vi "Actor Core.vi"(8 "error in":errorcluster, 11 "HIJ Vision Camera App In":refnum<class "HIJ Vision Camera App.lvclass">) -> (0 "error out":errorcluster, 3 "Actor out":refnum<class "Actor.lvclass">)   [LabVIEW 2014, in "HIJ Vision Camera App.lvlib" / "HIJ Vision Camera App.lvclass"]
doc: "(<B>Filename</B>: Actor Framework.lvlib:Actor.lvclass:Actor Core.vi)\n\nReceives messages to the actor, reacts to them, and initiates any error handling that may shut the actor down.\n\nDescendant classes may override this VI to append parallel tasks for the actor to complete while it handles messages. Overrides use the Call Parent Method node."
uses:
  HIJ Vision Camera App.lvclass
  <vilib>/ActorFramework/Actor/Actor.lvclass
  <vilib>/ActorFramework/Actor/Actor.lvclass/Actor.ctl
  <vilib>/ActorFramework/Message Enqueuer/Message Enqueuer.lvclass/Message Enqueuer.ctl
  HIJ Vision Camera App.lvclass/HIJ Vision Camera App.ctl
  HIJ Vision Camera App Dialog/HIJ Vision Camera App Dialog/HIJ Vision Camera App Dialog.lvclass/HIJ Vision Camera App Dialog.ctl
  HIJ Vision Application/HIJ Vision Application Messages/Write WorkDir Msg/Write WorkDir Msg.lvclass/Write WorkDir Msg.ctl
  HIJ Vision Camera App Messages/Write ConfigDir Msg/Write ConfigDir Msg.lvclass/Write ConfigDir Msg.ctl
  HIJ Vision Application/HIJ Vision Application Messages/Write Image Prefix Msg/Write Image Prefix Msg.lvclass/Write Image Prefix Msg.ctl
  HIJ Vision Camera App Messages/Start Aquisition Msg/Start Aquisition Msg.lvclass/Start Aquisition Msg.ctl
  Shared Code/Viewable Actor/ViewableActor Messages/Insert Into SubPanel Msg/Insert Into SubPanel Msg.lvclass/Insert Into SubPanel Msg.ctl
  HIJ Vision Camera App Dialog/HIJ Vision Camera App Dialog/Read Acquire.vi
  HIJ Vision Camera App Dialog/HIJ Vision Camera App Dialog/Read Camera Name.vi
  HIJ Vision Camera App Dialog/HIJ Vision Camera App Dialog/Read Prefix.vi
  HIJ Vision Camera App Dialog/HIJ Vision Camera App Dialog/Read ConfigDir.vi
  HIJ Vision Camera App Dialog/HIJ Vision Camera App Dialog/Read WorkDir.vi
  <vilib>/ActorFramework/Message Enqueuer/Init from Existing Queue.vi
  <vilib>/ActorFramework/Message Enqueuer/Enqueue.vi
  <vilib>/ActorFramework/Message Priority Queue/Priority Enqueue.vi
  <vilib>/ActorFramework/Message Enqueuer/Message Enqueuer.lvclass
  HIJ Vision Application/HIJ Vision Application Messages/Write WorkDir Msg/Write WorkDir Msg.lvclass
  HIJ Vision Camera App Messages/Write ConfigDir Msg/Write ConfigDir Msg.lvclass
  HIJ Vision Application/HIJ Vision Application Messages/Write Image Prefix Msg/Write Image Prefix Msg.lvclass
  HIJ Vision Camera App Messages/Start Aquisition Msg/Start Aquisition Msg.lvclass
  Shared Code/Viewable Actor/ViewableActor Messages/Insert Into SubPanel Msg/Insert Into SubPanel Msg.lvclass
  HIJ Vision Application/HIJ Vision Application/HIJ Vision Application.lvclass
  HIJ Vision Camera App Dialog/HIJ Vision Camera App Dialog/HIJ Vision Camera App Dialog.lvclass
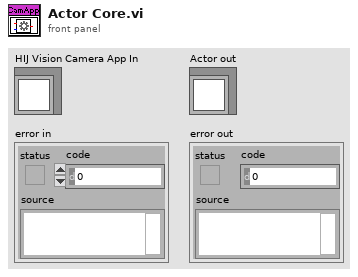
[diagram p1: front panel]
types:
  T1 = typedef "IMAQdx.ctl" = refnum<k21>
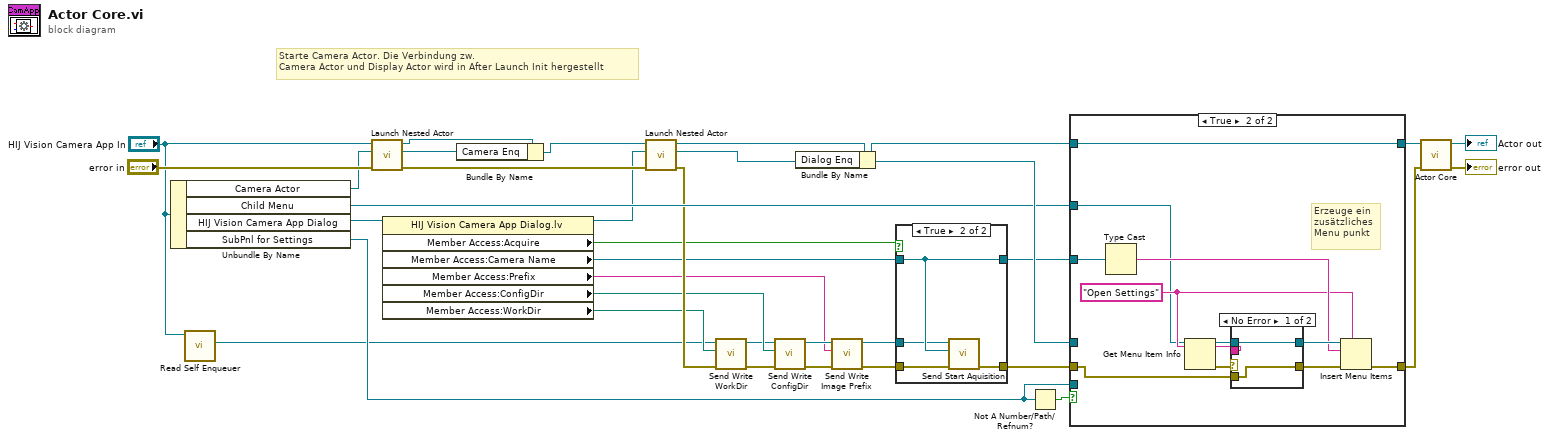
[diagram p0: block diagram]
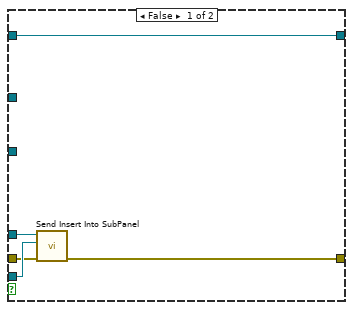
[diagram p3: hidden frame]
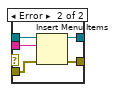
[diagram p4: hidden frame]
diagram:
  # "Starte Camera Actor. Die Verbindung zw.\nCamera Actor und Display Actor wird in After Launch Init hergestellt"
  n1 = Unbundle By Name("HIJ Vision Camera App In") -> ("Camera Actor"=w27:refnum<class "Camera Actor.lvclass">, "Child Menu"=w33:refnum<k9>, "HIJ Vision Camera App Dialog"=w23:refnum<class "HIJ Vision Camera App Dialog.lvclass">, "SubPnl for Settings"=w21:refnum<vi>)
  n2 = call <vilib>:"Read Self Enqueuer.vi"("Actor"="HIJ Vision Camera App In") -> ("Self Enqueuer"=w17:refnum<class "Message Enqueuer.lvclass">)  [unwired: 10 in]
  n3 = call <vilib>:"Launch Nested Actor.vi"("error in (no error)"="error in", "Nested Actor"=w27, "Caller Actor in"="HIJ Vision Camera App In") -> ("error out"=w24:errorcluster, "Nested Actor's Enqueuer"=w26:refnum<class "Message Enqueuer.lvclass">, "Caller Actor out"=w28:refnum<class "HIJ Vision Camera App.lvclass">)  [unwired: 6 in]
  n4 = property class="HIJ Vision Camera App Dialog.lv"(reference=w23) -> (reference out=w19:refnum<class "HIJ Vision Camera App Dialog.lvclass">, "Member Access:Acquire"=w8:bool, "Member Access:Camera Name"=w7:T1, "Member Access:Prefix"=w9:string, "Member Access:ConfigDir"=w16:path, "Member Access:WorkDir"=w18:path)  [unwired: 1 in, 1 out]
  n5 = Bundle By Name(cluster=w28, "Camera Enq"=w26) -> (w25:refnum<class "HIJ Vision Camera App.lvclass">)
  n6 = call <vilib>:"Launch Nested Actor.vi"("error in (no error)"=w24, "Nested Actor"=w19, "Caller Actor in"=w25) -> ("error out"=w32:errorcluster, "Nested Actor's Enqueuer"=w34:refnum<class "Message Enqueuer.lvclass">, "Caller Actor out"=w11:refnum<class "HIJ Vision Camera App.lvclass">)  [unwired: 6 in]
  n7 = call "Send Write WorkDir.vi"("error in (no error)"=w32, "Work Dir"=w18, "Message Enqueuer"=w17) -> ("error out"=w13:errorcluster, "Message Enqueuer out"=w15:refnum<class "Message Enqueuer.lvclass">)  [unwired: 7 in]
  n8 = call "Send Write ConfigDir.vi"("error in (no error)"=w13, "Work Dir"=w16, "Message Enqueuer"=w15) -> ("error out"=w12:errorcluster, "Message Enqueuer out"=w14:refnum<class "Message Enqueuer.lvclass">)  [unwired: 7 in]
  n9 = Bundle By Name(cluster=w11, "Dialog Enq"=w34) -> (w1:refnum<class "HIJ Vision Camera App.lvclass">)
  n10 = call "Send Write Image Prefix.vi"("error in (no error)"=w12, "Prefix"=w9, "Message Enqueuer"=w14) -> ("error out"=w5:errorcluster, "Message Enqueuer out"=w6:refnum<class "Message Enqueuer.lvclass">)  [unwired: 7 in]
  n11 = case shown="True" w8 {
    tunnel: w7 -> [w35 w40]
    tunnel: w6 -> [_ w39]
    tunnel: w5 -> [w36 w38]
    tunnel: [w36 w37] -> w4
    tunnel: [w35 w40] -> w3
    frame False {
    }
    frame True {
      n12 = call "Send Start Aquisition.vi"("error in (no error)"=w38, "Camera"=w40, "Message Enqueuer"=w39) -> ("error out"=w37:errorcluster)  [unwired: 7 in, 1 out]
    }
  }
  n13 = Not A Number/Path/Refnum?(number/path/refnum=w21) -> (NaN/Path/Refnum?=w22:bool)
  n14 = case shown="True" w22 {
    tunnel: w34 -> [w45 _]
    tunnel: w21 -> [w44 _]
    tunnel: w4 -> [w42 w46]
    tunnel: [w43 w55] -> w20
    tunnel: w33 -> [_ w49]
    tunnel: w3 -> [_ w53]
    tunnel: [w41 w51] -> w2
    tunnel: w1 -> [w41 w51]
    frame False {
      n15 = call "Send Insert Into SubPanel.vi"("error in (no error)"=w42, "SubPanel Ref"=w44, "Message Enqueuer"=w45) -> ("error out"=w43:errorcluster)  [unwired: 7 in, 1 out]
    }
    frame True {
      w50 = "Open Settings"
      # "Erzeuge ein \nzusätzliches \nMenu punkt"
      n16 = Type Cast(x=w53) -> (*(type *) &x=w52:string)  [unwired: 1 in]
      n17 = Get Menu Item Info(7:w50, 11:w49) -> (0:w47:errorcluster, 3:w48:refnum<k9>)  [unwired: 1 in, 5 out]
      n18 = case shown="No Error" w47 {
        tunnel: [w57 w63] -> w56
        tunnel: [w58 w62] -> w54
        tunnel: w50 -> [_ w61]
        tunnel: w48 -> [w58 w60]
        tunnel: w46 -> [w57 w59]
        frame No Error {
        }
        frame Error {
          n19 = Insert Menu Items(6:w59, 8:w61, 9:w60) -> (0:w63:errorcluster, 3:w62:refnum<k9>)  [unwired: 3 in, 1 out]
        }
      }
      n20 = Insert Menu Items(5:w50, 6:w56, 8:w52, 9:w54) -> (0:w55:errorcluster)  [unwired: 2 in, 2 out]
    }
  }
  n21 = call-parent "Actor Core.vi"("error in"=w20, "Launch IMAQ Display in"=w2) -> ("error out"=→"error out":errorcluster, "Actor out"=→"Actor out":refnum<class "Actor.lvclass">)  [unwired: 8 in]
